vi "RR autofocus.vi"(0 "Close camera shutter during autofocus?":bool=TRUE, 2 "Close laser shutter when autofocus is done?":bool=TRUE) -> (6 "error out":errorcluster caption="Errors/Warnings")   [LabVIEW 2016]
doc: "Uses quandrant photodiode to to retroreflection autofocus based on previously stored calibration table."
uses:
  Stage/Move stage command.ctl
  Autofocus Globals.vi
  newhnu shutters/hardware status globals.vi
  <vilib>/Analysis/NI_AALBase.lvlib
  <vilib>/Analysis/NI_AALPro.lvlib
panel:
  out "Delta z":dbl
  out "Power":dbl
  out "Calibration curve and fit":cluster{"QPD position":dbl[], "z (um)":ext[]}[](graph)
  in  "error in":errorcluster
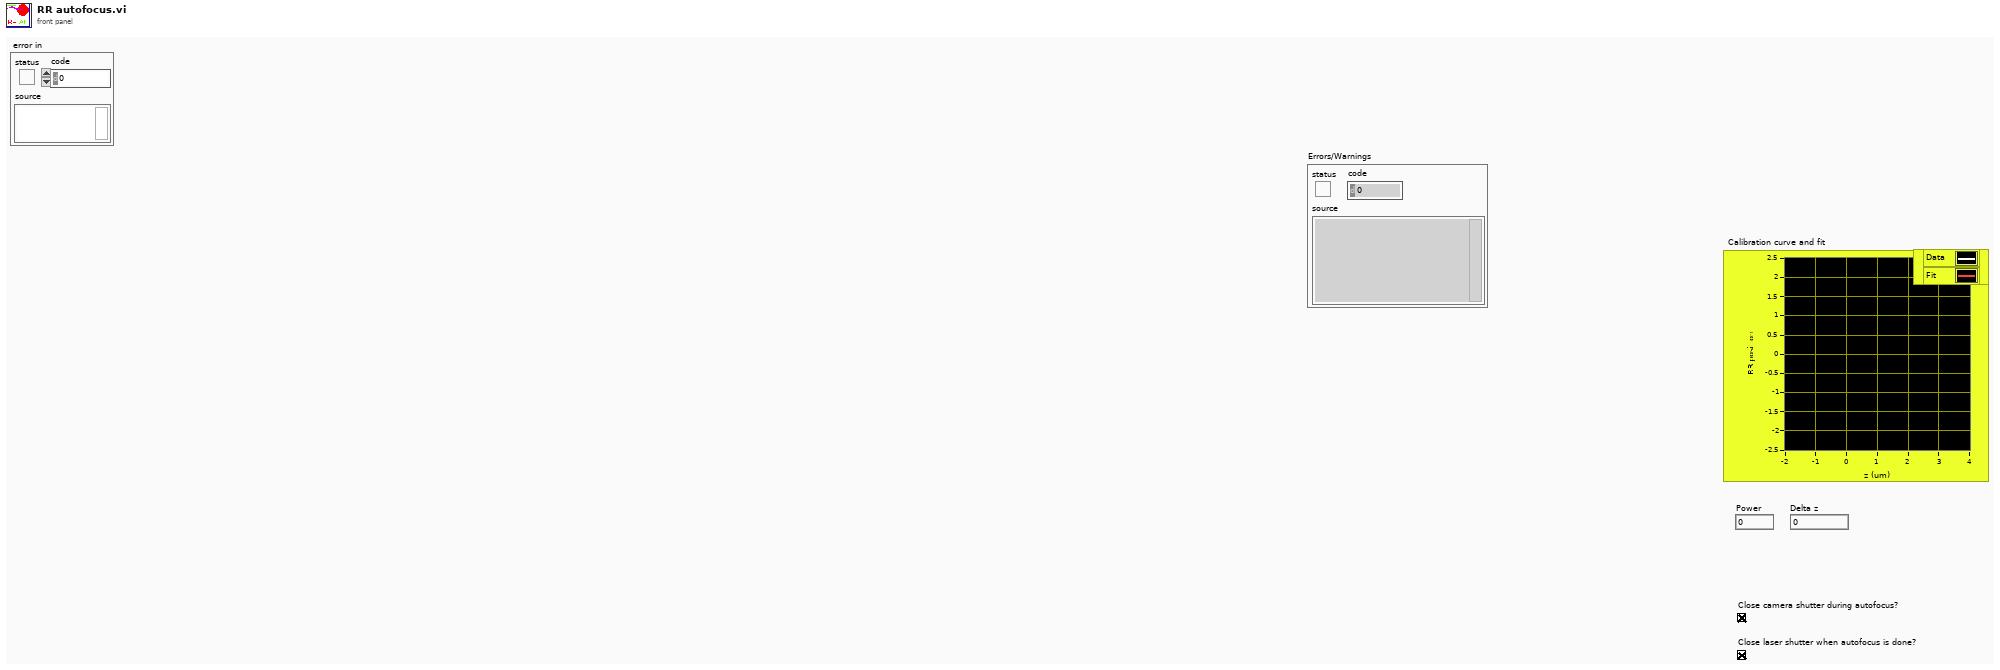
[diagram p1: front panel]
types:
  T1 = typedef "Move stage command.ctl" = cluster{"dx (um) (0 -> ignore)":ext, "dy (um) (0 -> ignore)":ext, "dz (um) (0 -> ignore)":ext, "Re-center x,y":bool, "Re-center z":bool, "x (um) (-1 -> ignore)":dbl, "y (um) (-1 -> ignore)":dbl, "z (um) (-1 -> ignore)":dbl}
  T2 = typedef "Laser type.ctt" = enum16{"Blue 488 nm", "Green 532 nm", "Red 635 nm", "IR 785"}
  T3 = cluster{"QPD position":dbl[], "Best Polynomial Fit":dbl[]}
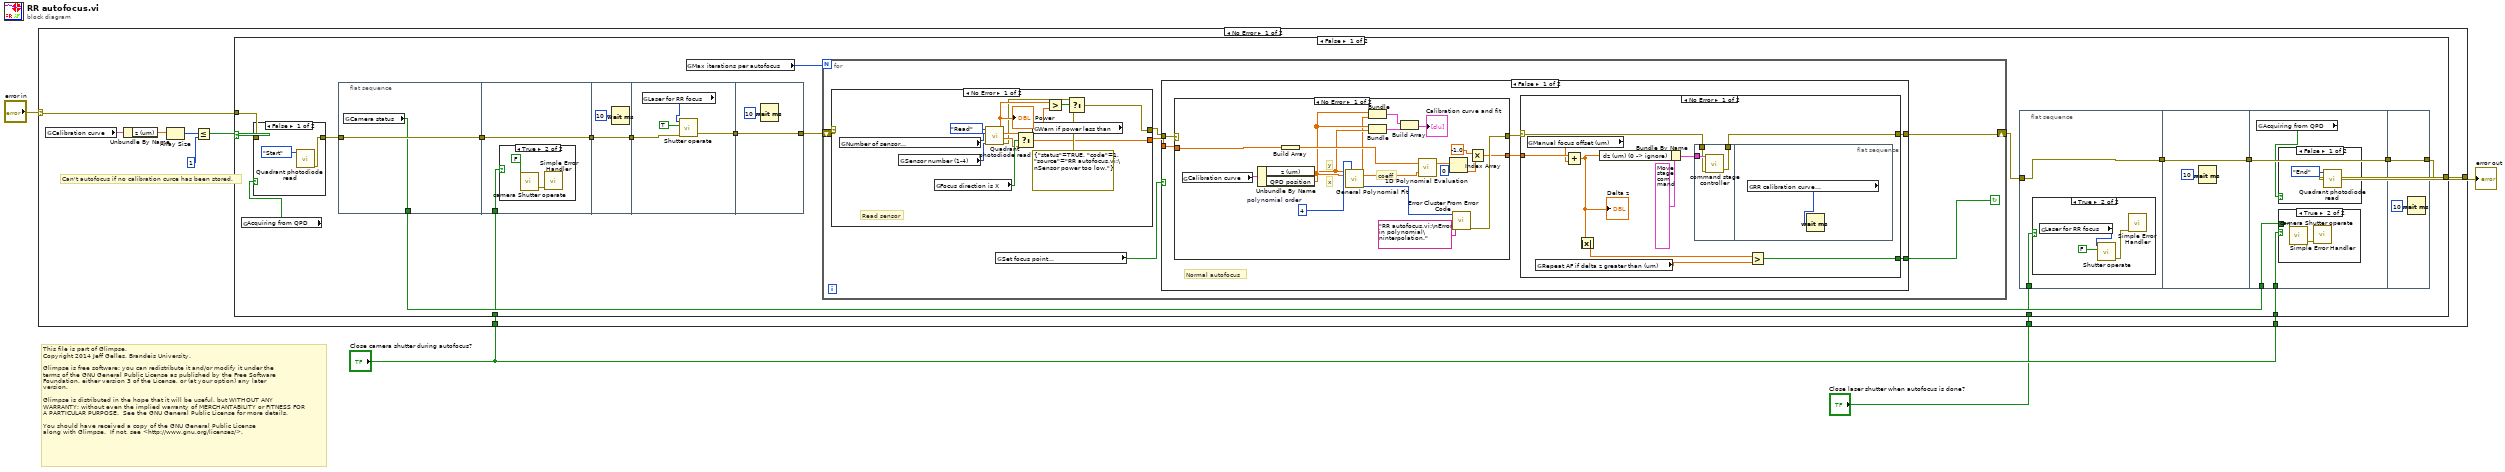
[diagram p0: block diagram]
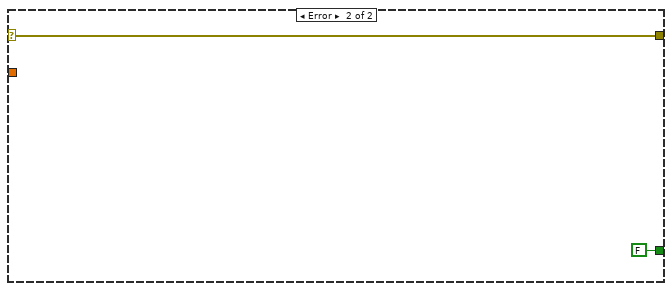
[diagram p2: hidden frame]
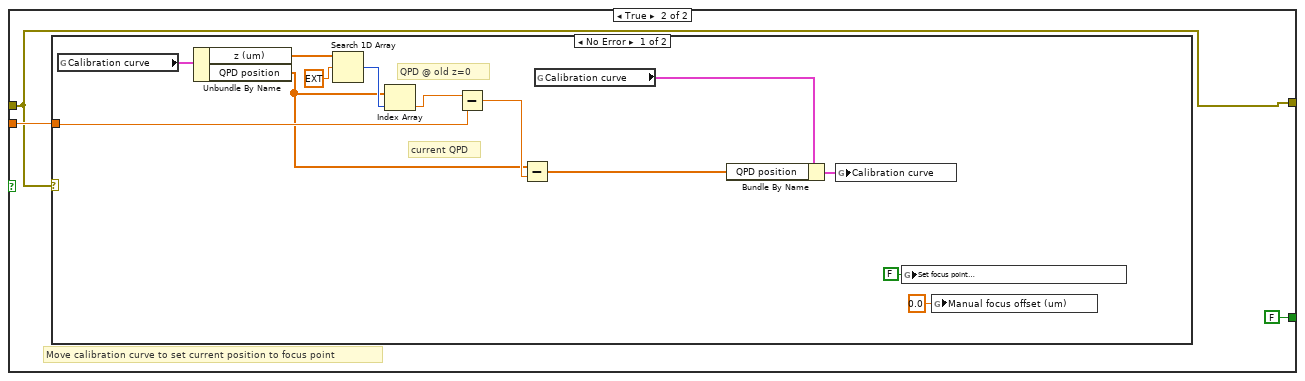
[diagram p4: hidden frame]
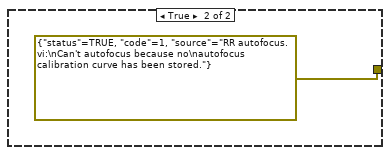
[diagram p12: hidden frame]
diagram:
  # "This file is part of Glimpse. \nCopyright 2014 Jeff Gelles, Brandeis University.    \n\nGlimpse is free software: you can redistribute it and/or modify it under the \nterms of the GNU General Public License as published by the Free Software \nFoundation, either version 3 of the License, or (at your option) any later \nversion.\n\nGlimpse is distributed in the hope that it will be useful, but WITHOUT ANY \nWARRANTY; without even the implied warranty of MERCHANTABILITY or FITNESS FOR \nA PARTICULAR PURPOSE.  See the GNU General Public License for more details.\n\nYou should have received a copy of the GNU General Public License\nalong with Glimpse.  If not, see <http://www.gnu.org/licenses/>."
  n1 = case shown="No Error" "error in" {
    selector: "error in" -> [w14 w146]
    tunnel: [w13 w146] -> w3
    tunnel: "Close camera shutter during autofocus?" -> [w7 _]
    tunnel: "Close camera shutter during autofocus?" -> [w6 _]
    tunnel: "Close laser shutter when autofocus is done?" -> [w5 _]
    frame No Error {
      # "Can't autofocus if no calibration curce has been stored."
      n2 = global read "Autofocus Globals.vi" "Calibration curve"() -> (w12:cluster{"z (um)":ext[], "QPD position":dbl[]})
      n3 = Unbundle By Name(w12) -> ("z (um)"=w11:ext[])
      n4 = Array Size(array=w11) -> (size(s)=w10:i32)
      n5 = Less Or Equal?(x=w10, y=1) -> (x <= y?=w8:bool)
      n6 = case shown="False" w8 {
        tunnel: w14 -> [w26 _]
        tunnel: [w22 errorcluster {"status"=TRUE, "code"=1, "source"="RR autofocus.vi:\nCan't autofocus because no\nautofocus calibration curve has been stored."} ("f")] -> w13
        tunnel: w7 -> [w19 _]
        tunnel: w6 -> [w18 _]
        tunnel: w5 -> [w17 _]
        frame False {
          n7 = global read "Autofocus Globals.vi" "Acquiring from QPD"() -> (w25:bool)
          n8 = case shown="False" w25 {
            tunnel: w26 -> [_ w144]
            tunnel: [w142 w144] -> w24
            frame False {
              n9 = call "Quadrant photodiode read.vi"("Mode"=enum16{"Start", "Read", "End"}."Start") -> ("error out"=w142:errorcluster)  [unwired: 2 in, 6 out]
            }
            frame True {
            }
          }
          n10 = flat-sequence {
            tunnel: w24 -> [w129]
            tunnel: [w129] -> w21
            tunnel: [w128] -> w20
            tunnel: [w131] -> w32
            tunnel: w21 -> [w131]
            tunnel: w19 -> [w130]
            tunnel: w32 -> [w135]
            tunnel: [w135] -> w31
            tunnel: [w136] -> w30
            tunnel: w31 -> [w137]
            tunnel: [w141] -> w23
            tunnel: w30 -> [w141]
            frame #0 {
              n11 = global read "hardware status globals.vi" "Camera status"() -> (w128:bool)
            }
            frame #1 {
              n12 = case shown="True" w130 {
                frame False {
                }
                frame True {
                  n13 = call "camera Shutter operate.vi"("Open?"=FALSE) -> ("error out"=w132:errorcluster)  [unwired: 1 in, 6 out]
                  n14 = call <vilib>:"Simple Error Handler.vi"("error in (no error)"=w132) -> ()  [unwired: 1 in, 8 out]
                }
              }
            }
            frame #2 {
              n15 = Wait (ms)(milliseconds to wait=u32 10) -> ()  [unwired: 1 out]
            }
            frame #3 {
              n16 = global read "Autofocus Globals.vi" "Laser for RR focus"() -> (w138:T2[])
              n17 = call "Shutter operate.vi"("Shutters"=w138, 2:TRUE ("Data to Write"), "error in"=w137) -> ("error out"=w136:errorcluster)  [unwired: 5 out]
            }
            frame #4 {
              n18 = Wait (ms)(milliseconds to wait=u32 10) -> ()  [unwired: 1 out]
            }
          }
          n19 = global read "Autofocus Globals.vi" "Max iterations per autofocus"() -> (w15:i32)
          n20 = for {
            N: w15 -> [_]
            shift-right: [w34] -> w16
            shift-left: w23 -> [w36]
            stop <- w33 continue-if-true
            n21 = case shown="No Error" w36 {
              selector: w36 -> [_ w111]
              tunnel: [w100 w111] -> w38
              tunnel: [w99 _] -> w37
              frame No Error {
                # "Read sensor"
                n22 = global read "Autofocus Globals.vi" "Number of sensor\nreadings to average"() -> (w98:i32)
                n23 = global read "Autofocus Globals.vi" "Sensor number (1-4)"() -> (w109:i8)
                n24 = global read "Autofocus Globals.vi" "Focus direction is X"() -> (w108:bool)
                n25 = call "Quadrant photodiode read.vi"("Sensor Number\n(ignored)"=w109, "number of readings\n to average"=w98, "Mode"=enum16{"Start", "Read", "End"}."Read") -> ("error out"=w102:errorcluster, "Y position"=w104:dbl, "X position"=w105:dbl, "Power"=w106:dbl)  [unwired: 3 out]
                "Power" <- w106
                n26 = Select(t=w105, s=w108, f=w104) -> (s? t:f=w99:dbl)
                n27 = global read "Autofocus Globals.vi" "Warn if power less than"() -> (w107:dbl)
                n28 = Greater?(x=w106, y=w107) -> (0:w103:bool)
                n29 = Select(t=w102, s=w103, f=errorcluster {"status"=TRUE, "code"=1, "source"="RR autofocus.vi:\nSensor power too low."}) -> (s? t:f=w100:errorcluster)
              }
              frame Error {
              }
            }
            n30 = global read "Autofocus Globals.vi" "Set focus point\nto current z position"() -> (w35:bool)
            n31 = case shown="False" w35 {
              tunnel: w38 -> [w44 w83]
              tunnel: w37 -> [w43 w84]
              tunnel: [w40 w83] -> w34
              tunnel: [w39 FALSE] -> w33
              frame False {
                # "Normal autofocus"
                n32 = case shown="No Error" w44 {
                  selector: w44 -> [_ w81]
                  tunnel: w43 -> [w73 w80]
                  tunnel: [w75 w81] -> w42
                  tunnel: [w68 w80] -> w41
                  frame No Error {
                    w67 = 4  # polynomial order
                    # "coeff"
                    # "y"
                    # "x"
                    n33 = global read "Autofocus Globals.vi" "Calibration curve"() -> (w79:cluster{"z (um)":ext[], "QPD position":dbl[]})
                    n34 = Unbundle By Name(w79) -> ("z (um)"=w64:ext[], "QPD position"=w65:dbl[])
                    n35 = Build Array(w73) -> (w72:dbl[])
                    n36 = call <vilib>:"General Polynomial Fit.vi"("Y"=w64, "polynomial order"=w67, "X"=w65) -> ("Best Polynomial Fit"=w63:dbl[], "Polynomial Coefficients"=w74:dbl[], "error"=w78:i32)  [unwired: 9 in, 1 out]
                    n37 = Bundle("QPD position"=w65, "Best Polynomial Fit"=w63) -> (w62:T3)  [unwired: 1 out]
                    n38 = Bundle("QPD position"=w65, "z (um)"=w64) -> (w61:cluster{"QPD position":dbl[], "z (um)":ext[]})  [unwired: 1 out]
                    n39 = Build Array(w62, w61) -> (→"Calibration curve and fit":cluster{"QPD position":dbl[], "z (um)":ext[]}[])
                    n40 = call <vilib>:"1D Polynomial Evaluation.vi"("Coefficients: a"=w74, "X"=w72) -> ("Y"=w71:dbl[])  [unwired: 1 out]
                    n41 = Index Array(array=w71, index=0) -> (element=w69:dbl)
                    n42 = call <vilib>:"Error Cluster From Error Code.vi"("error message (\"\")"="RR autofocus.vi:\nError in polynomial\ninterpolation." ("error message (\"\")"), "error code (0)"=w78) -> ("error out"=w75:errorcluster)  [unwired: 2 in, 5 out]
                    n43 = Multiply(x=-1.0, y=w69) -> (x*y=w68:dbl)
                  }
                  frame Error {
                  }
                }
                n44 = case shown="No Error" w42 {
                  selector: w42 -> [w51 w60]
                  tunnel: w41 -> [w53 _]
                  tunnel: [w50 w60] -> w40
                  tunnel: [w47 FALSE] -> w39
                  frame No Error {
                    n45 = global read "Autofocus Globals.vi" "Manual focus offset (um)"() -> (w49:dbl)
                    n46 = global read "Autofocus Globals.vi" "Repeat AF if delta z greater than (um)"() -> (w46:dbl)
                    n47 = Add(x=w53, y=w49) -> (x+y=w48:dbl)
                    "Delta z" <- w48
                    n48 = Absolute Value(x=w48) -> (abs(x)=w45:dbl)
                    n49 = Bundle By Name(cluster=T1 {"dx (um) (0 -> ignore)"=0.0, "dy (um) (0 -> ignore)"=0.0, "dz (um) (0 -> ignore)"=0.0, "Re-center x,y"=FALSE, "Re-center z"=FALSE, "x (um) (-1 -> ignore)"=-1.0, "y (um) (-1 -> ignore)"=-1.0, "z (um) (-1 -> ignore)"=-1.0} ("command"), "dz (um) (0 -> ignore)"=w48) -> (w54:T1)
                    n50 = flat-sequence {
                      tunnel: w54 -> [w57]
                      tunnel: w51 -> [w56]
                      tunnel: [w55] -> w50
                      frame #0 {
                        n51 = call "command stage controller.vi"("command"=w57, "error in (no error)"=w56) -> ("error out"=w55:errorcluster)  [unwired: 6 out]
                      }
                      frame #1 {
                        n52 = global read "Autofocus Globals.vi" "RR calibration curve\nsettle time (ms)"() -> (w58:u16)
                        n53 = Wait (ms)(milliseconds to wait=w58) -> ()  [unwired: 1 out]
                      }
                    }
                    n54 = Greater?(x=w45, y=w46) -> (0:w47:bool)
                  }
                  frame Error {
                  }
                }
              }
              frame True {
                # "Move calibration curve to set current position to focus point"
                n55 = case shown="No Error" w83 {
                  tunnel: w84 -> [w94 _]
                  frame No Error {
                    # "current QPD"
                    # "QPD @ old z=0"
                    n56 = global read "Autofocus Globals.vi" "Calibration curve"() -> (w97:cluster{"z (um)":ext[], "QPD position":dbl[]})
                    n57 = Unbundle By Name(w97) -> ("z (um)"=w92:ext[], "QPD position"=w86:dbl[])
                    n58 = Search 1D Array(1D array=w92, element=ext 0.0) -> (index of element=w95:i32)  [unwired: 1 in]
                    n59 = Index Array(array=w86, index=w95) -> (element=w93:dbl)
                    n60 = Subtract(x=w93, y=w94) -> (x-y=w91:dbl)
                    n61 = Subtract(x=w86, y=w91) -> (x-y=w88:dbl[])
                    n62 = global read "Autofocus Globals.vi" "Calibration curve"() -> (w89:cluster{"z (um)":ext[], "QPD position":dbl[]})
                    n63 = Bundle By Name(cluster=w89, "QPD position"=w88) -> (w90:cluster{"z (um)":ext[], "QPD position":dbl[]})
                    n64 = global write "Autofocus Globals.vi" "Calibration curve"(w90) -> ()
                    n65 = global write "Autofocus Globals.vi" "Set focus point\nto current z position"(FALSE ("Set current z position to focus point")) -> ()
                    n66 = global write "Autofocus Globals.vi" "Manual focus offset (um)"(0.0 ("Manual focus offset (um)")) -> ()
                  }
                  frame Error {
                  }
                }
              }
            }
          }
          n67 = flat-sequence {
            tunnel: w16 -> [w113]
            tunnel: [w113] -> w29
            tunnel: w17 -> [w112]
            tunnel: w29 -> [w117]
            tunnel: [w117] -> w28
            tunnel: w28 -> [w122]
            tunnel: [w122] -> w27
            tunnel: w20 -> [w120]
            tunnel: w18 -> [w119]
            tunnel: [w127] -> w22
            tunnel: w27 -> [w127]
            frame #0 {
              n68 = case shown="True" w112 {
                frame False {
                }
                frame True {
                  n69 = global read "Autofocus Globals.vi" "Laser for RR focus"() -> (w115:T2[])
                  n70 = call "Shutter operate.vi"("Shutters"=w115, 2:FALSE ("Data to Write")) -> ("error out"=w114:errorcluster)  [unwired: 1 in, 5 out]
                  n71 = call <vilib>:"Simple Error Handler.vi"("error in (no error)"=w114) -> ()  [unwired: 1 in, 8 out]
                }
              }
            }
            frame #1 {
              n72 = Wait (ms)(milliseconds to wait=u32 10) -> ()  [unwired: 1 out]
            }
            frame #2 {
              n73 = global read "Autofocus Globals.vi" "Acquiring from QPD"() -> (w121:bool)
              n74 = case shown="False" w121 {
                frame False {
                  n75 = call "Quadrant photodiode read.vi"("Mode"=enum16{"Start", "Read", "End"}."End") -> ()  [unwired: 2 in, 7 out]
                }
                frame True {
                }
              }
              n76 = case shown="True" w119 {
                tunnel: w120 -> [_ w123]
                frame False {
                }
                frame True {
                  n77 = call "camera Shutter operate.vi"("Open?"=w123) -> ("error out"=w124:errorcluster)  [unwired: 1 in, 6 out]
                  n78 = call <vilib>:"Simple Error Handler.vi"("error in (no error)"=w124) -> ()  [unwired: 1 in, 8 out]
                }
              }
            }
            frame #3 {
              n79 = Wait (ms)(milliseconds to wait=u32 10) -> ()  [unwired: 1 out]
            }
          }
        }
        frame True {
        }
      }
    }
    frame Error {
      # "error"
    }
  }
  "error out" <- w3
